vi "Begin.vi"(8 "error in":errorcluster) -> (0 "error out":errorcluster)   [LabVIEW 2018]
doc: "Called before other user functions, this VI is expected to open initial I/O refnums, load in file data, and do all program initialization. Notice that the <B>error out</B> terminal is simply used for data flow. Wiring it to other structures or subVIs ensures that this VI runs first."
uses:
  <vilib>/Rock Robotics/WPI/DriverStation/WPI_DriverStationRobotMode2.ctl
  <vilib>/Rock Robotics/WPI/Joystick/WPI_JoystickDeviceEnum.ctl
  <vilib>/Rock Robotics/WPI/ThirdParty/Phoenix-LabVIEW/Motor Controller/Controls/CTRE_Phoenix_MotorControl_ControlMode.ctl
  <vilib>/Rock Robotics/WPI/ThirdParty/Phoenix-LabVIEW/Motor Controller/Controls/CTRE_Phoenix_MotorControl_NeutralMode.ctl
  <vilib>/Rock Robotics/WPI/ThirdParty/Phoenix-LabVIEW/Motor Controller/Controls/CTRE_Phoenix_MotorControl_FeedbackDevice.ctl
  <vilib>/Rock Robotics/WPI/Solenoid/WPI_SolenoidChannel.ctl
  <vilib>/Rock Robotics/SystemInterfaces/DIO/FPGA_DIOChannel.ctl
  <vilib>/Rock Robotics/SystemInterfaces/AI/FPGA_AIChannel.ctl
  Robot Global Data.vi
  <vilib>/Rock Robotics/Network Tables/NT Write Numeric Array.vi
  <vilib>/Rock Robotics/WPI/Utilities/WPI_GetSetVariantRefNum.vi
  <vilib>/Rock Robotics/WPI/Solenoid/WPI_SolenoidOpenDouble.vi
  <vilib>/Rock Robotics/WPI/Ultrasonic/WPI_SonarMB1010AnalogOpen.vi
  <vilib>/Rock Robotics/WPI/Ultrasonic/WPI_SonarMB1010AnalogRefNum Registry Set.vi
  <vilib>/Rock Robotics/Network Tables/NT Write String Array.vi
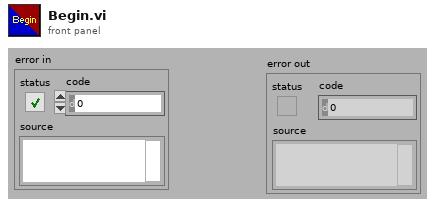
[diagram p1: front panel]
types:
  T1 = typedef "FPGA_DIOChannel.ctl" = enum8{"DIO 0", "DIO 1", "DIO 2", "DIO 3", "DIO 4", "DIO 5", "DIO 6", "DIO 7", "DIO 8", "DIO 9", "DIO MXP 0", "DIO MXP 1", "DIO MXP 2", "DIO MXP 3", "DIO MXP 4", "DIO MXP 5", "DIO MXP 6", "DIO MXP 7", "DIO MXP 8", "DIO MXP 9", "DIO MXP 10", "DIO MXP 11", "DIO MXP 12", "DIO MXP 13", "DIO MXP 14", "DIO MXP 15", "SPI Port CS1", "SPI Port CS2", "SPI Port CS3", "SPI Port MISO", "SPI Port MOSI", "Invalid"}
  T2 = typedef "FPGA_AIChannel.ctl" = enum8{"AI 0", "AI 1", "AI 2", "AI 3", "AI MXP 0", "AI MXP 1", "AI MXP 2", "AI MXP 3", "Invalid"}
  T3 = typedef "WPI_SolenoidChannel.ctl" = enum8{"Solenoid 0", "Solenoid 1", "Solenoid 2", "Solenoid 3", "Solenoid 4", "Solenoid 5", "Solenoid 6", "Solenoid 7", "Invalid"}
  T4 = typedef "CTRE_Phoenix_MotorControl_FeedbackDevice.ctl" = i8
  T5 = typedef "CTRE_Phoenix_MotorControl_NeutralMode.ctl" = enum8{"EEPROMSetting", "Override to Coast", "Override to Brake"}
  T6 = typedef "CTRE_Phoenix_MotorControl_ControlMode.ctl" = u16
  T7 = typedef "WPI_JoystickDeviceEnum.ctl" = enum16{"USB 0", "USB 1", "USB 2", "USB 3", "USB 4", "USB 5"}
  T8 = typedef "WPI_DriverStationRobotMode2.ctl" = enum16{"Autonomous Disabled", "Autonomous Enabled", "Teleop Disabled", "Teleop Enabled", "Disconnected", "Finish", "Test Disabled", "Test Enabled", "Emergency Stopped"}
  T9 = typedef "WPI_JoystickDevRef.ctl" = cluster{"Device":T7}
  T10 = typedef "WPI_DigitalInputDevRef.ctl" = cluster{"DevStatus":errorcluster, "DIO Channel":T1}
  T11 = typedef "WPI_MotorControlDeviceRef.ctl" = cluster{"DeviceStatus":errorcluster, "Type":T12, "PWM":cluster{"PWM Channel":T13, "DeadBand":T14}, "CAN":cluster{"Device Number":u8, "SetOutput VI Ref":variant, "GetOutput VI Ref":variant, "Enable VI Ref":variant, "Disable VI Ref":variant, "Data":variant}, "Invert":bool, "DIO PWM":cluster{"PWM \"Enable\" Channel":T13, "DIOChannel":T1, "PWM Rate":dbl}}
  T12 = typedef "WPI_MotorControlType.ctl" = enum16{"PWM", "CAN", "DIO PWM"}
  T13 = typedef "FPGA_DIOPWMChannel.ctl" = enum8{"PWM 0", "PWM 1", "PWM 2", "PWM 3", "PWM 4", "PWM 5", "PWM 6", "PWM 7", "PWM 8", "PWM 9", "PWM MXP 0", "PWM MXP 1", "PWM MXP 2", "PWM MXP 3", "PWM MXP 4", "PWM MXP 5", "PWM MXP 6", "PWM MXP 7", "PWM MXP 8", "PWM MXP 9", "Invalid"}
  T14 = typedef "WPI_PWMDeadband.ctl" = cluster{"Name":string, "maxPositivePwm":i32, "minPositivePwm":i32, "centerPwm":i32, "maxNegativePwm":i32, "minNegativePwm":i32, "angularRange":u16}
  T15 = typedef "WPI_CompressorDevRef.ctl" = cluster{"DevStatus":errorcluster, "Pneumatics Control Module":u8}
  T16 = typedef "WPI_SolenoidDevRef.ctl" = cluster{"DevStatus":errorcluster, "Pneumatics Control Module":u8, "Forward Solenoid Channel":T3, "Reverse Solenoid Channel":T3}
  T17 = typedef "WPI_SonarMB1010AnalogDeviceRef.ctl" = cluster{"AIDeviceRef":T18, "Scaling factor (V/in)":dbl, "Average Bits":u8}
  T18 = typedef "WPI_AnalogChannelDevRef.ctl" = cluster{"DevStatus":errorcluster, "Analog Channel":T2}
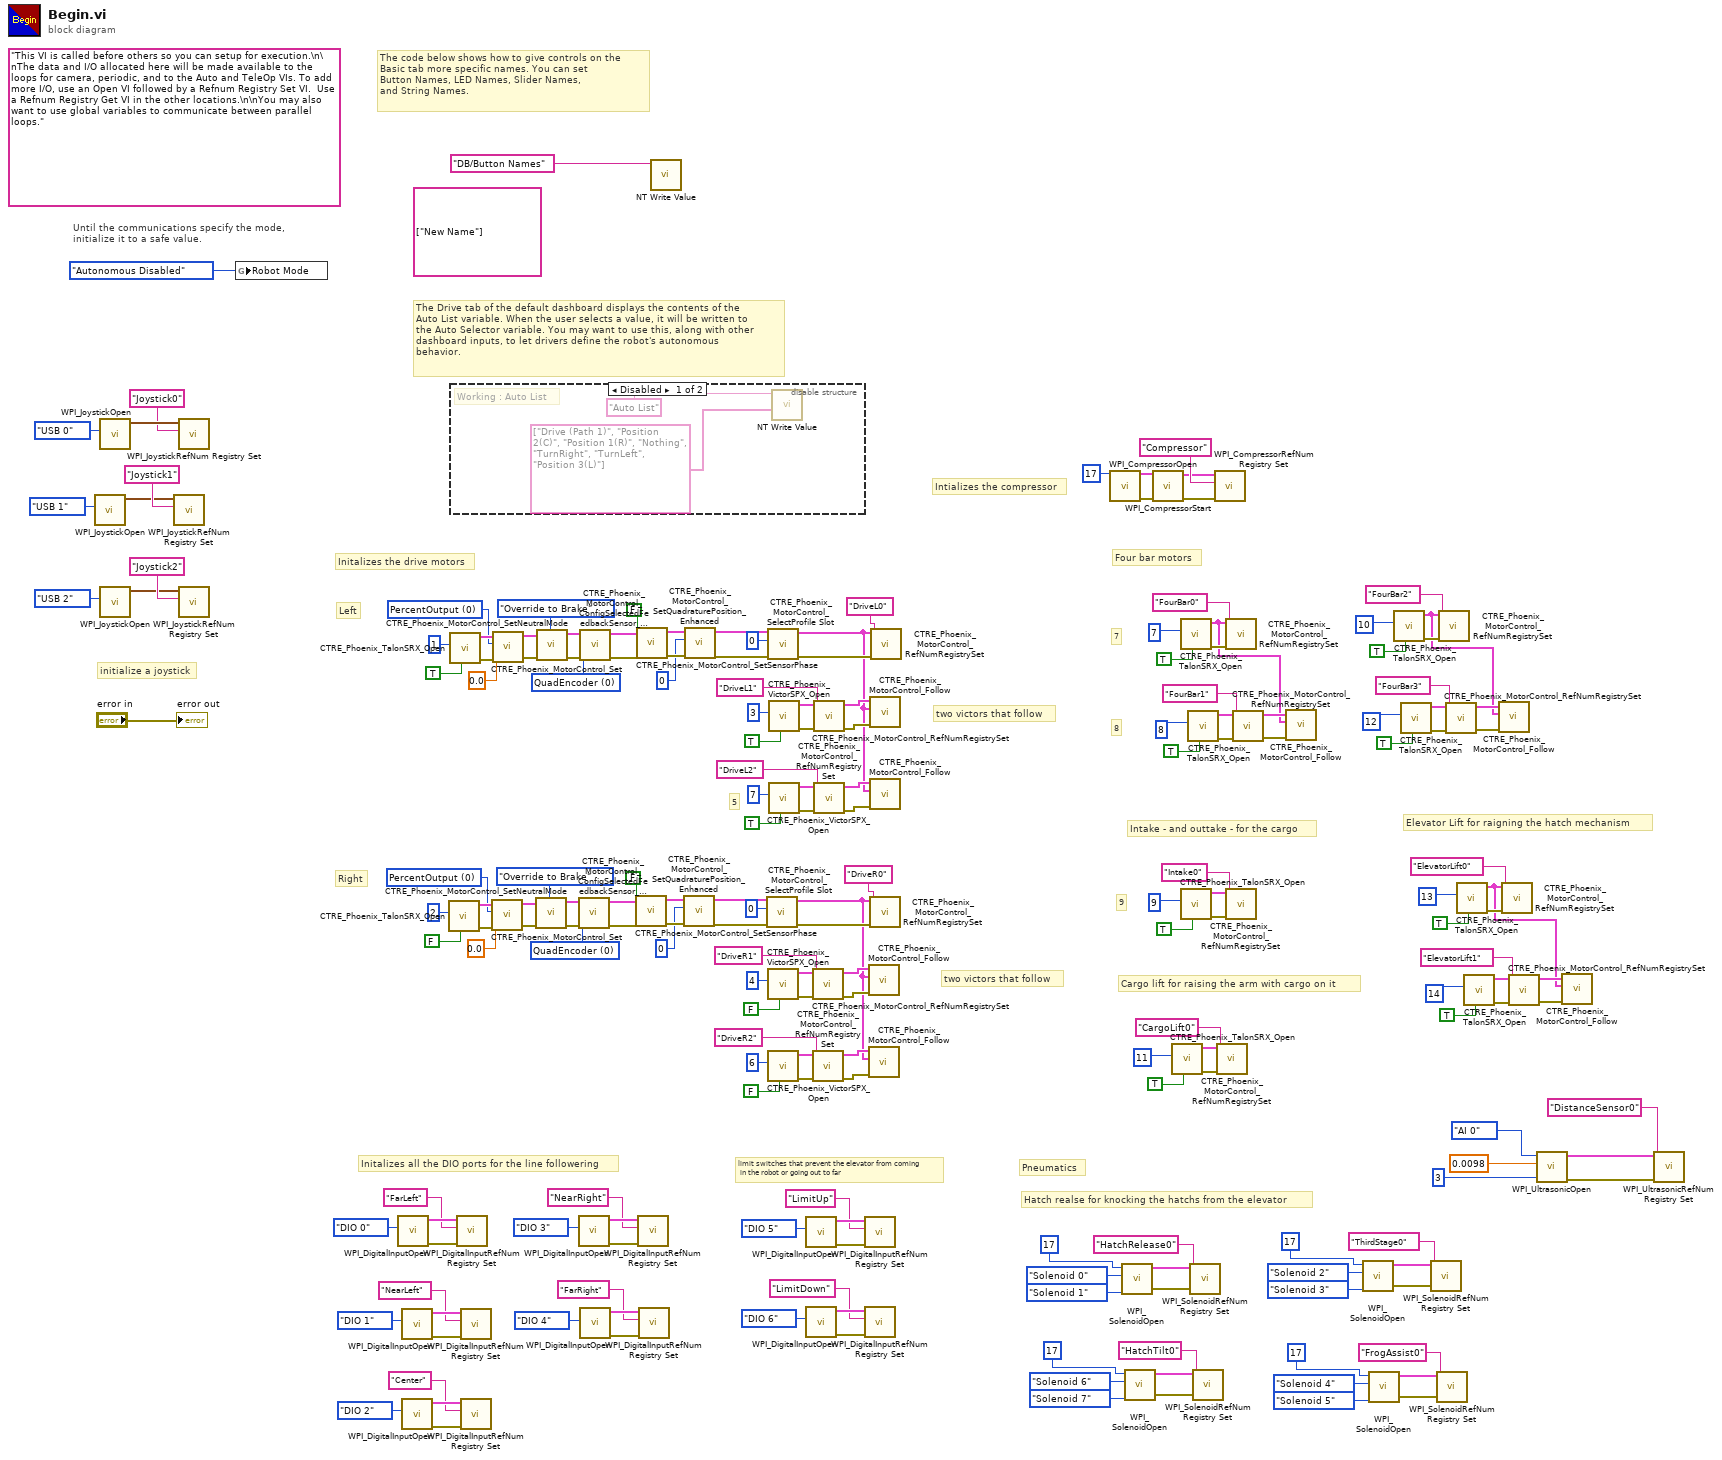
[diagram p0: block diagram]
diagram:
  w115 = T4 0 items=["None"=-1, "QuadEncoder"=0, "Analog"=2, "Tachometer"=4, "Pulse Width Encoded Position"=8, "Sensor Sum (S0 + S1)"=9, "Sensor Difference (D0 - D1)"=10, "Remote Source 0"=11, "Remote Source 1"=12, "Software Emulated"=15] ("Feedback Device")
  w120 = T6 0 items=["PercentOutput"=0, "Position"=1, "Velocity"=2, "Current"=3, "Follower"=5, "MotionProfile"=6, "MotionMagic"=7, "MotionMagicArc"=8, "MotionProfileArc"=10, "Disabled"=15] ("Control Mode")
  w153 = T4 0 items=["None"=-1, "QuadEncoder"=0, "Analog"=2, "Tachometer"=4, "Pulse Width Encoded Position"=8, "Sensor Sum (S0 + S1)"=9, "Sensor Difference (D0 - D1)"=10, "Remote Source 0"=11, "Remote Source 1"=12, "Software Emulated"=15] ("Feedback Device")
  w158 = T6 0 items=["PercentOutput"=0, "Position"=1, "Velocity"=2, "Current"=3, "Follower"=5, "MotionProfile"=6, "MotionMagic"=7, "MotionMagicArc"=8, "MotionProfileArc"=10, "Disabled"=15] ("Control Mode")
  (unwired) string[] ["New Name"]
  (unwired) "This VI is called before others so you can setup for execution.\n\nThe data and I/O allocated here will be made available to the loops for camera, periodic, and to the Auto and TeleOp VIs. To add more I/O, use an Open VI followed by a Refnum Registry Set VI.  Use a Refnum Registry Get VI in the other locations.\n\nYou may also want to use global variables to communicate between parallel loops."
  # "limit switches that prevent the elevator from coming\n in the robot or going out to far"
  # "9"
  # "5"
  # "8"
  # "7"
  # "Hatch realse for knocking the hatchs from the elevator"
  # "Pneumatics"
  # "Initalizes all the DIO ports for the line followering"
  # "Intializes the compressor"
  # "Elevator Lift for raigning the hatch mechanism"
  # "Cargo lift for raising the arm with cargo on it"
  # "Intake - and outtake - for the cargo"
  # "Four bar motors"
  # "two victors that follow"
  # "two victors that follow"
  # "Right"
  # "Left"
  # "Initalizes the drive motors"
  # "The Drive tab of the default dashboard displays the contents of the\nAuto List variable. When the user selects a value, it will be written to\nthe Auto Selector variable. You may want to use this, along with other\ndashboard inputs, to let drivers define the robot's autonomous\nbehavior."
  # "The code below shows how to give controls on the\nBasic tab more specific names. You can set\nButton Names, LED Names, Slider Names,\nand String Names."
  # "initialize a joystick"
  # "Until the communications specify the mode,\ninitialize it to a safe value."
  n1 = call <vilib>:"WPI_JoystickOpen.vi"("JoystickDevice"=WPI_JoystickDeviceEnum."USB 1") -> ("JoystickDevRef"=w196:T9)  [unwired: 10 in]
  n2 = call <vilib>:"WPI_JoystickOpen.vi"("JoystickDevice"=WPI_JoystickDeviceEnum."USB 0") -> ("JoystickDevRef"=w191:T9)  [unwired: 10 in]
  n3 = call <vilib>:"WPI_JoystickOpen.vi"("JoystickDevice"=WPI_JoystickDeviceEnum."USB 2") -> ("JoystickDevRef"=w188:T9)  [unwired: 10 in]
  n4 = call <vilib>:"WPI_JoystickRefNum Registry Set.vi"("refnum name"="Joystick1", "JoystickDevRef"=w196) -> ()  [unwired: 8 in, 2 out]
  n5 = call <vilib>:"WPI_JoystickRefNum Registry Set.vi"("refnum name"="Joystick0", "JoystickDevRef"=w191) -> ()  [unwired: 8 in, 2 out]
  n6 = call <vilib>:"WPI_JoystickRefNum Registry Set.vi"("refnum name"="Joystick2", "JoystickDevRef"=w188) -> ()  [unwired: 8 in, 2 out]
  n7 = global write "Robot Global Data.vi" "Robot Mode"(WPI_DriverStationRobotMode2."Autonomous Disabled" ("Robot Mode")) -> ()
  n8 = call <vilib>:"WPI_DigitalInputOpen.vi"("DIO Channel"=FPGA_DIOChannel."DIO 0") -> ("error out"=w71:errorcluster, "DigitalInputDevRef"=w70:T10)  [unwired: 9 in]
  n9 = call <vilib>:"WPI_DigitalInputOpen.vi"("DIO Channel"=FPGA_DIOChannel."DIO 1") -> ("error out"=w68:errorcluster, "DigitalInputDevRef"=w67:T10)  [unwired: 9 in]
  n10 = call <vilib>:"WPI_DigitalInputOpen.vi"("DIO Channel"=FPGA_DIOChannel."DIO 2") -> ("error out"=w65:errorcluster, "DigitalInputDevRef"=w64:T10)  [unwired: 9 in]
  n11 = call "CTRE_Phoenix_TalonSRX_Open.vi"("Invert"=FALSE, "Device Number"=u8 2) -> ("error out"=w123:errorcluster, "CAN Talon SRX Ref"=w124:T11)  [unwired: 8 in]
  n12 = call "CTRE_Phoenix_TalonSRX_Open.vi"("Invert"=TRUE, "Device Number"=u8 1) -> ("error out"=w161:errorcluster, "CAN Talon SRX Ref"=w162:T11)  [unwired: 8 in]
  n13 = disable-structure shown="Disabled" {
    frame Disabled {
      # "Working : Auto List"
      n14 = call-poly <vilib>:"NT Write Value.vi"("String Array"=string[] ["Drive (Path 1)", "Position 2(C)", "Position 1(R)", "Nothing", "TurnRight", "TurnLeft", "Position 3(L)"], "Name"="Auto List") -> ()  [unwired: 9 in, 1 out]
    }
    frame Enabled {
    }
  }
  n15 = call <vilib>:"WPI_DigitalInputRefNum Registry Set.vi"("error in (no error)"=w71, "refnum name"="FarLeft", "DigitalInputDevRef"=w70) -> ()  [unwired: 7 in, 2 out]
  n16 = call <vilib>:"WPI_DigitalInputRefNum Registry Set.vi"("error in (no error)"=w68, "refnum name"="NearLeft", "DigitalInputDevRef"=w67) -> ()  [unwired: 7 in, 2 out]
  n17 = call <vilib>:"WPI_DigitalInputRefNum Registry Set.vi"("error in (no error)"=w65, "refnum name"="Center", "DigitalInputDevRef"=w64) -> ()  [unwired: 7 in, 2 out]
  n18 = call <vilib>:"CTRE_Phoenix_MotorControl_Set.vi"("error in (no error)"=w123, "Output"=0.0, "Control Mode"=w120, "PhoenixMotorControlDevRef"=w124) -> ("error out"=w121:errorcluster, "PhoenixMotorControlDevRef"=w122:T11)  [unwired: 6 in]
  n19 = call <vilib>:"CTRE_Phoenix_MotorControl_Set.vi"("error in (no error)"=w161, "Output"=0.0, "Control Mode"=w158, "PhoenixMotorControlDevRef"=w162) -> ("error out"=w159:errorcluster, "PhoenixMotorControlDevRef"=w160:T11)  [unwired: 6 in]
  n20 = call <vilib>:"CTRE_Phoenix_MotorControl_SetNeutralMode.vi"("error in (no error)"=w121, "Motor Control Neutral Mode"=CTRE_Phoenix_MotorControl_NeutralMode."Override to Brake", "PhoenixMotorControlDevRef"=w122) -> ("error out"=w117:errorcluster, "PhoenixMotorControlDevRef"=w116:T11)  [unwired: 7 in]
  n21 = call <vilib>:"CTRE_Phoenix_MotorControl_SetNeutralMode.vi"("error in (no error)"=w159, "Motor Control Neutral Mode"=CTRE_Phoenix_MotorControl_NeutralMode."Override to Brake", "PhoenixMotorControlDevRef"=w160) -> ("error out"=w155:errorcluster, "PhoenixMotorControlDevRef"=w154:T11)  [unwired: 7 in]
  n22 = call <vilib>:"CTRE_Phoenix_MotorControl_ConfigSelectedFeedbackSensor_Enhanced.vi"("error in (no error)"=w117, "Feedback Device"=w115, "PhoenixMotorControlDevRef"=w116) -> ("error out"=w113:errorcluster, "PhoenixMotorControlDevRef"=w114:T11)  [unwired: 7 in]
  n23 = call <vilib>:"WPI_DigitalInputOpen.vi"("DIO Channel"=FPGA_DIOChannel."DIO 3") -> ("error out"=w62:errorcluster, "DigitalInputDevRef"=w61:T10)  [unwired: 9 in]
  n24 = call <vilib>:"CTRE_Phoenix_MotorControl_ConfigSelectedFeedbackSensor_Enhanced.vi"("error in (no error)"=w155, "Feedback Device"=w153, "PhoenixMotorControlDevRef"=w154) -> ("error out"=w151:errorcluster, "PhoenixMotorControlDevRef"=w152:T11)  [unwired: 7 in]
  n25 = call <vilib>:"WPI_DigitalInputOpen.vi"("DIO Channel"=FPGA_DIOChannel."DIO 4") -> ("error out"=w59:errorcluster, "DigitalInputDevRef"=w58:T10)  [unwired: 9 in]
  n26 = call <vilib>:"CTRE_Phoenix_MotorControl_SetSensorPhase.vi"("error in (no error)"=w113, "PhaseSensor"=FALSE, "PhoenixMotorControlDevRef"=w114) -> ("error out"=w111:errorcluster, "PhoenixMotorControlDevRef"=w110:T11)  [unwired: 7 in]
  n27 = call <vilib>:"CTRE_Phoenix_MotorControl_SetSensorPhase.vi"("error in (no error)"=w151, "PhaseSensor"=FALSE, "PhoenixMotorControlDevRef"=w152) -> ("error out"=w149:errorcluster, "PhoenixMotorControlDevRef"=w148:T11)  [unwired: 7 in]
  n28 = call <vilib>:"WPI_DigitalInputRefNum Registry Set.vi"("error in (no error)"=w62, "refnum name"="NearRight", "DigitalInputDevRef"=w61) -> ()  [unwired: 7 in, 2 out]
  n29 = call <vilib>:"WPI_DigitalInputRefNum Registry Set.vi"("error in (no error)"=w59, "refnum name"="FarRight", "DigitalInputDevRef"=w58) -> ()  [unwired: 7 in, 2 out]
  n30 = call-poly <vilib>:"NT Write Value.vi"("Name"="DB/Button Names") -> ()  [unwired: 10 in, 1 out]
  n31 = call <vilib>:"CTRE_Phoenix_MotorControl_SetQuadraturePosition_Enhanced.vi"("error in (no error)"=w111, "New Position"=0, "PhoenixMotorControlDevRef"=w110) -> ("error out"=w105:errorcluster, "PhoenixMotorControlDevRef"=w106:T11)  [unwired: 7 in]
  n32 = call <vilib>:"CTRE_Phoenix_MotorControl_SetQuadraturePosition_Enhanced.vi"("error in (no error)"=w149, "New Position"=0, "PhoenixMotorControlDevRef"=w148) -> ("error out"=w143:errorcluster, "PhoenixMotorControlDevRef"=w144:T11)  [unwired: 7 in]
  n33 = call <vilib>:"CTRE_Phoenix_MotorControl_SelectProfile Slot.vi"("error in (no error)"=w105, "slotIdx"=0, "PhoenixMotorControlDevRef"=w106) -> ("error out"=w108:errorcluster, "PhoenixMotorControlDevRef"=w97:T11)  [unwired: 7 in]
  n34 = call <vilib>:"CTRE_Phoenix_MotorControl_SelectProfile Slot.vi"("error in (no error)"=w143, "slotIdx"=0, "PhoenixMotorControlDevRef"=w144) -> ("error out"=w146:errorcluster, "PhoenixMotorControlDevRef"=w135:T11)  [unwired: 7 in]
  n35 = call <vilib>:"CTRE_Phoenix_VictorSPX_Open.vi"("Invert"=FALSE, "Device Number"=u8 4) -> ("error out"=w131:errorcluster, "CAN Talon SRX Ref"=w130:T11)  [unwired: 8 in]
  n36 = call <vilib>:"CTRE_Phoenix_VictorSPX_Open.vi"("Invert"=FALSE, "Device Number"=u8 6) -> ("error out"=w103:errorcluster, "CAN Talon SRX Ref"=w102:T11)  [unwired: 8 in]
  n37 = call <vilib>:"CTRE_Phoenix_VictorSPX_Open.vi"("Invert"=TRUE, "Device Number"=u8 3) -> ("error out"=w169:errorcluster, "CAN Talon SRX Ref"=w168:T11)  [unwired: 8 in]
  n38 = call <vilib>:"CTRE_Phoenix_VictorSPX_Open.vi"("Invert"=TRUE, "Device Number"=u8 7) -> ("error out"=w141:errorcluster, "CAN Talon SRX Ref"=w140:T11)  [unwired: 8 in]
  n39 = call <vilib>:"WPI_DigitalInputOpen.vi"("DIO Channel"=FPGA_DIOChannel."DIO 5") -> ("error out"=w8:errorcluster, "DigitalInputDevRef"=w7:T10)  [unwired: 9 in]
  n40 = call <vilib>:"WPI_DigitalInputOpen.vi"("DIO Channel"=FPGA_DIOChannel."DIO 6") -> ("error out"=w5:errorcluster, "DigitalInputDevRef"=w4:T10)  [unwired: 9 in]
  n41 = call <vilib>:"CTRE_Phoenix_MotorControl_RefNumRegistrySet.vi"("error in (no error)"=w131, "refnum name"="DriveR1", "PhoenixMotorControlDevRef"=w130) -> ("error out"=w128:errorcluster, "PhoenixMotorControlDevRef"=w127:T11)  [unwired: 7 in]
  n42 = call <vilib>:"CTRE_Phoenix_MotorControl_RefNumRegistrySet.vi"("error in (no error)"=w103, "refnum name"="DriveR2", "PhoenixMotorControlDevRef"=w102) -> ("error out"=w100:errorcluster, "PhoenixMotorControlDevRef"=w99:T11)  [unwired: 7 in]
  n43 = call <vilib>:"CTRE_Phoenix_MotorControl_RefNumRegistrySet.vi"("error in (no error)"=w169, "refnum name"="DriveL1", "PhoenixMotorControlDevRef"=w168) -> ("error out"=w166:errorcluster, "PhoenixMotorControlDevRef"=w165:T11)  [unwired: 7 in]
  n44 = call <vilib>:"CTRE_Phoenix_MotorControl_RefNumRegistrySet.vi"("error in (no error)"=w141, "refnum name"="DriveL2", "PhoenixMotorControlDevRef"=w140) -> ("error out"=w138:errorcluster, "PhoenixMotorControlDevRef"=w137:T11)  [unwired: 7 in]
  n45 = call <vilib>:"WPI_DigitalInputRefNum Registry Set.vi"("error in (no error)"=w8, "refnum name"="LimitUp", "DigitalInputDevRef"=w7) -> ()  [unwired: 7 in, 2 out]
  n46 = call <vilib>:"WPI_DigitalInputRefNum Registry Set.vi"("error in (no error)"=w5, "refnum name"="LimitDown", "DigitalInputDevRef"=w4) -> ()  [unwired: 7 in, 2 out]
  n47 = call <vilib>:"CTRE_Phoenix_MotorControl_Follow.vi"("error in (no error)"=w128, "Master Controller to Follow"=w97, "PhoenixMotorControlDevRef"=w127) -> ()  [unwired: 7 in, 2 out]
  n48 = call <vilib>:"CTRE_Phoenix_MotorControl_Follow.vi"("error in (no error)"=w100, "Master Controller to Follow"=w97, "PhoenixMotorControlDevRef"=w99) -> ()  [unwired: 7 in, 2 out]
  n49 = call <vilib>:"CTRE_Phoenix_MotorControl_Follow.vi"("error in (no error)"=w166, "Master Controller to Follow"=w135, "PhoenixMotorControlDevRef"=w165) -> ()  [unwired: 7 in, 2 out]
  n50 = call <vilib>:"CTRE_Phoenix_MotorControl_Follow.vi"("error in (no error)"=w138, "Master Controller to Follow"=w135, "PhoenixMotorControlDevRef"=w137) -> ()  [unwired: 7 in, 2 out]
  n51 = call <vilib>:"CTRE_Phoenix_MotorControl_RefNumRegistrySet.vi"("error in (no error)"=w108, "refnum name"="DriveR0", "PhoenixMotorControlDevRef"=w97) -> ()  [unwired: 7 in, 2 out]
  n52 = call <vilib>:"CTRE_Phoenix_MotorControl_RefNumRegistrySet.vi"("error in (no error)"=w146, "refnum name"="DriveL0", "PhoenixMotorControlDevRef"=w135) -> ()  [unwired: 7 in, 2 out]
  n53 = call <vilib>:"WPI_CompressorOpen.vi"("Pneumatics Control Module (0)"=u8 17) -> ("CompressorDevRef"=w185:T15, "error out"=w184:errorcluster)  [unwired: 13 in]
  n54 = call-poly <vilib>:"WPI_SolenoidOpen.vi"("Reverse Solenoid Channel"=WPI_SolenoidChannel."Solenoid 1", "Forward Solenoid Channel"=WPI_SolenoidChannel."Solenoid 0", "Pneumatics Control Module (0)"=u8 17) -> ("error out"=w56:errorcluster, "SolenoidDevRef"=w55:T16)  [unwired: 7 in]
  n55 = call-poly <vilib>:"WPI_SolenoidOpen.vi"("Reverse Solenoid Channel"=WPI_SolenoidChannel."Solenoid 7", "Forward Solenoid Channel"=WPI_SolenoidChannel."Solenoid 6", "Pneumatics Control Module (0)"=u8 17) -> ("error out"=w44:errorcluster, "SolenoidDevRef"=w43:T16)  [unwired: 7 in]
  n56 = call <vilib>:"WPI_CompressorStart.vi"("error in (no error)"=w184, "CompressorDevRef"=w185) -> ("error out"=w182:errorcluster, "CompressorDevRef"=w183:T15)  [unwired: 8 in]
  n57 = call "CTRE_Phoenix_TalonSRX_Open.vi"("Invert"=TRUE, "Device Number"=u8 11) -> ("error out"=w88:errorcluster, "CAN Talon SRX Ref"=w84:T11)  [unwired: 8 in]
  n58 = call "CTRE_Phoenix_TalonSRX_Open.vi"("Invert"=TRUE, "Device Number"=u8 7) -> ("error out"=w180:errorcluster, "CAN Talon SRX Ref"=w94:T11)  [unwired: 8 in]
  n59 = call "CTRE_Phoenix_TalonSRX_Open.vi"("Invert"=TRUE, "Device Number"=u8 9) -> ("error out"=w93:errorcluster, "CAN Talon SRX Ref"=w89:T11)  [unwired: 8 in]
  n60 = call "CTRE_Phoenix_TalonSRX_Open.vi"("Invert"=TRUE, "Device Number"=u8 8) -> ("error out"=w177:errorcluster, "CAN Talon SRX Ref"=w176:T11)  [unwired: 8 in]
  n61 = call <vilib>:"WPI_SolenoidRefNum Registry Set.vi"("error in (no error)"=w56, "refnum name"="HatchRelease0", "SolenoidDevRef"=w55) -> ()  [unwired: 7 in, 2 out]
  n62 = call <vilib>:"WPI_SolenoidRefNum Registry Set.vi"("error in (no error)"=w44, "refnum name"="HatchTilt0", "SolenoidDevRef"=w43) -> ()  [unwired: 7 in, 2 out]
  n63 = call <vilib>:"WPI_CompressorRefNum Registry Set.vi"("error in (no error)"=w182, "refnum name"="Compressor", "CompressorDevRef"=w183) -> ()  [unwired: 7 in, 2 out]
  n64 = call <vilib>:"CTRE_Phoenix_MotorControl_RefNumRegistrySet.vi"("error in (no error)"=w88, "refnum name"="CargoLift0", "PhoenixMotorControlDevRef"=w84) -> ()  [unwired: 7 in, 2 out]
  n65 = call <vilib>:"CTRE_Phoenix_MotorControl_RefNumRegistrySet.vi"("error in (no error)"=w180, "refnum name"="FourBar0", "PhoenixMotorControlDevRef"=w94) -> ()  [unwired: 7 in, 2 out]
  n66 = call <vilib>:"CTRE_Phoenix_MotorControl_RefNumRegistrySet.vi"("error in (no error)"=w93, "refnum name"="Intake0", "PhoenixMotorControlDevRef"=w89) -> ()  [unwired: 7 in, 2 out]
  n67 = call <vilib>:"CTRE_Phoenix_MotorControl_RefNumRegistrySet.vi"("error in (no error)"=w177, "refnum name"="FourBar1", "PhoenixMotorControlDevRef"=w176) -> ("error out"=w95:errorcluster, "PhoenixMotorControlDevRef"=w96:T11)  [unwired: 7 in]
  n68 = call <vilib>:"CTRE_Phoenix_MotorControl_Follow.vi"("error in (no error)"=w95, "Master Controller to Follow"=w94, "PhoenixMotorControlDevRef"=w96) -> ()  [unwired: 7 in, 2 out]
  n69 = call-poly <vilib>:"WPI_SolenoidOpen.vi"("Reverse Solenoid Channel"=WPI_SolenoidChannel."Solenoid 3", "Forward Solenoid Channel"=WPI_SolenoidChannel."Solenoid 2", "Pneumatics Control Module (0)"=u8 17) -> ("error out"=w38:errorcluster, "SolenoidDevRef"=w37:T16)  [unwired: 7 in]
  n70 = call-poly <vilib>:"WPI_SolenoidOpen.vi"("Reverse Solenoid Channel"=WPI_SolenoidChannel."Solenoid 5", "Forward Solenoid Channel"=WPI_SolenoidChannel."Solenoid 4", "Pneumatics Control Module (0)"=u8 17) -> ("error out"=w32:errorcluster, "SolenoidDevRef"=w31:T16)  [unwired: 7 in]
  n71 = call "CTRE_Phoenix_TalonSRX_Open.vi"("Invert"=TRUE, "Device Number"=u8 10) -> ("error out"=w26:errorcluster, "CAN Talon SRX Ref"=w16:T11)  [unwired: 8 in]
  n72 = call "CTRE_Phoenix_TalonSRX_Open.vi"("Invert"=TRUE, "Device Number"=u8 12) -> ("error out"=w23:errorcluster, "CAN Talon SRX Ref"=w22:T11)  [unwired: 8 in]
  n73 = call <vilib>:"WPI_SolenoidRefNum Registry Set.vi"("error in (no error)"=w38, "refnum name"="ThirdStage0", "SolenoidDevRef"=w37) -> ()  [unwired: 7 in, 2 out]
  n74 = call <vilib>:"WPI_SolenoidRefNum Registry Set.vi"("error in (no error)"=w32, "refnum name"="FrogAssist0", "SolenoidDevRef"=w31) -> ()  [unwired: 7 in, 2 out]
  n75 = call <vilib>:"CTRE_Phoenix_MotorControl_RefNumRegistrySet.vi"("error in (no error)"=w26, "refnum name"="FourBar2", "PhoenixMotorControlDevRef"=w16) -> ()  [unwired: 7 in, 2 out]
  n76 = call <vilib>:"CTRE_Phoenix_MotorControl_RefNumRegistrySet.vi"("error in (no error)"=w23, "refnum name"="FourBar3", "PhoenixMotorControlDevRef"=w22) -> ("error out"=w17:errorcluster, "PhoenixMotorControlDevRef"=w18:T11)  [unwired: 7 in]
  n77 = call "CTRE_Phoenix_TalonSRX_Open.vi"("Invert"=TRUE, "Device Number"=u8 13) -> ("error out"=w83:errorcluster, "CAN Talon SRX Ref"=w72:T11)  [unwired: 8 in]
  n78 = call "CTRE_Phoenix_TalonSRX_Open.vi"("Invert"=TRUE, "Device Number"=u8 14) -> ("error out"=w80:errorcluster, "CAN Talon SRX Ref"=w79:T11)  [unwired: 8 in]
  n79 = call <vilib>:"CTRE_Phoenix_MotorControl_Follow.vi"("error in (no error)"=w17, "Master Controller to Follow"=w16, "PhoenixMotorControlDevRef"=w18) -> ()  [unwired: 7 in, 2 out]
  n80 = call <vilib>:"CTRE_Phoenix_MotorControl_RefNumRegistrySet.vi"("error in (no error)"=w83, "refnum name"="ElevatorLift0", "PhoenixMotorControlDevRef"=w72) -> ()  [unwired: 7 in, 2 out]
  n81 = call <vilib>:"CTRE_Phoenix_MotorControl_RefNumRegistrySet.vi"("error in (no error)"=w80, "refnum name"="ElevatorLift1", "PhoenixMotorControlDevRef"=w79) -> ("error out"=w73:errorcluster, "PhoenixMotorControlDevRef"=w74:T11)  [unwired: 7 in]
  n82 = call-poly <vilib>:"WPI_UltrasonicOpen.vi"("Average Bits"=u8 3, "Scaling factor (V/in)"=0.0098, "Analog Channel"=FPGA_AIChannel."AI 0") -> ("error out"=w10:errorcluster, "SonarMB1010AnalogDevRef"=w11:T17)  [unwired: 7 in]
  n83 = call <vilib>:"CTRE_Phoenix_MotorControl_Follow.vi"("error in (no error)"=w73, "Master Controller to Follow"=w72, "PhoenixMotorControlDevRef"=w74) -> ()  [unwired: 7 in, 2 out]
  n84 = call-poly <vilib>:"WPI_UltrasonicRefNum Registry Set.vi"("error in (no error)"=w10, "refnum name"="DistanceSensor0", "SonarMB1010AnalogDevRef"=w11) -> ()  [unwired: 7 in, 2 out]
  "error out" <- "error in"
